vi "Save Snapshot.vi"(6 "IPath Getter in":refnum<class "IPath Getter.lvclass">, 8 "error in":errorcluster, 10 "Debug Elements Options":T1={"Breakpoints"=TRUE, "Probes"=TRUE}, 11 "VI Reference in":refnum<vi>) -> (0 "error out":errorcluster, 3 "VI Reference out":refnum<vi>)   [LabVIEW 2020, in "Public API.lvlib"]
doc: "Save <b>Debug Snapshot</b> (i.e. breakpoints and probes) of the active VI."
uses:
  Public API.lvlib
  Type Definitions/Snapshot Handling Options--cluster.ctl
  IPath Getter/IPath Getter.lvclass
  Type Definitions/Class Name--enum.ctl
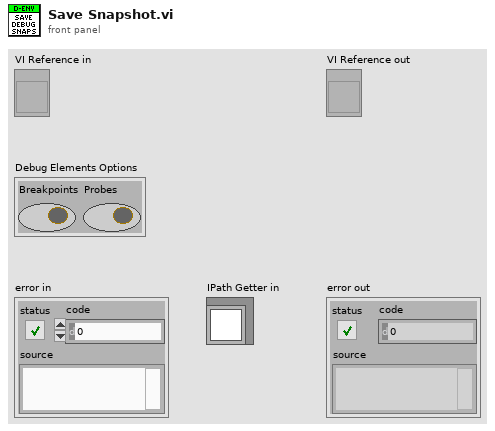
[diagram p1: front panel]
types:
  T1 = typedef "Snapshot Handling Options--cluster.ctl" = cluster{"Breakpoints":bool, "Probes":bool}
  T2 = typedef "Class Name--enum.ctl" = enum16{"Node", "Wire"}
  T3 = typedef "Breakpoint--cluster.ctl" = cluster{"UID":i32, "BP Status":T4, "Class Name":T2}
  T4 = typedef "LVBreakpointStatusEnum.ctl" = enum8{"Cleared Break", "Enabled Break", "Disabled Break"}
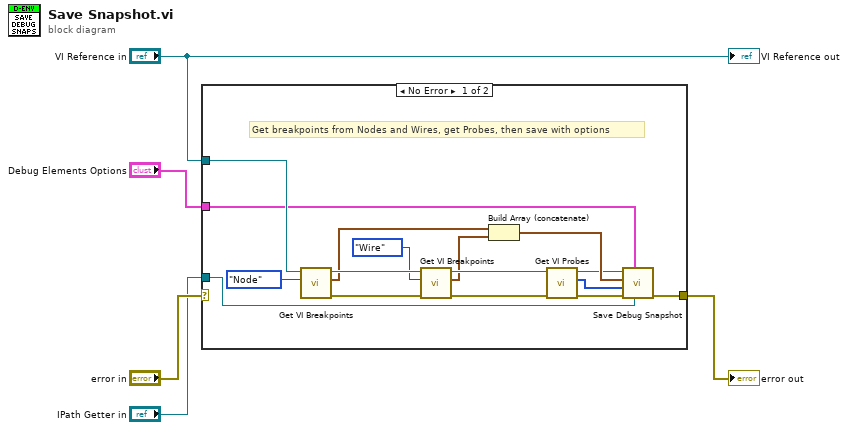
[diagram p0: block diagram]
diagram:
  n1 = case shown="No Error" "error in" {
    selector: "error in" -> [_ w22]
    tunnel: "VI Reference in" -> [w17 _]
    tunnel: "Debug Elements Options" -> [w7 _]
    tunnel: [w18 w22] -> w4
    tunnel: "IPath Getter in" -> [w6 _]
    frame No Error {
      # "Get breakpoints from Nodes and Wires, get Probes, then save with options"
      n2 = call "Get VI Breakpoints.vi"("Class Name"=Class_Name--enum."Node", "VI Reference in"=w17) -> ("error out"=w21:errorcluster, "Breakpoints"=w12:T3[], "VI Reference out"=w16:refnum<vi>)  [unwired: 7 in]
      n3 = call "Get VI Breakpoints.vi"("error in"=w21, "Class Name"=Class_Name--enum."Wire", "VI Reference in"=w16) -> ("error out"=w20:errorcluster, "Breakpoints"=w11:T3[], "VI Reference out"=w15:refnum<vi>)  [unwired: 6 in]
      n4 = Build Array (concatenate)(w12, w11) -> (w10:T3[])
      n5 = call "Get VI Probes.vi"("error in"=w20, "VI Reference in"=w15) -> ("error out"=w19:errorcluster, "Probes"=w9:i32[], "VI Reference out"=w8:refnum<vi>)  [unwired: 7 in]
      n6 = call "Save Debug Snapshot.vi"("IPath Getter in"=w6, "Debug Elements Options"=w7, "error in"=w19, "Probes"=w9, "Breakpoints"=w10, "VI Reference in"=w8) -> ("error out"=w18:errorcluster)  [unwired: 4 in, 1 out]
    }
    frame Error {
      # "Pass error without further action"
    }
  }
  "error out" <- w4
  "VI Reference out" <- "VI Reference in"
